vi "Fade Overlay.vi"(11 "Stop Fade":refnum<user-event>) -> ()   [LabVIEW 2020]
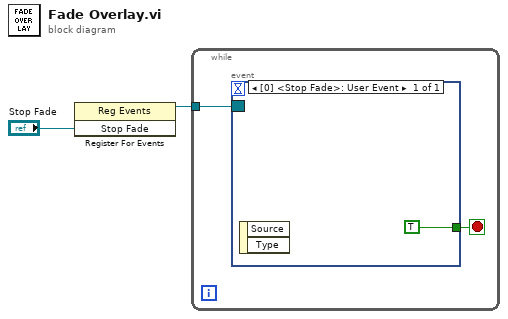
[diagram p0: block diagram]
diagram:
  n1 = register-events("Stop Fade") -> (reference out=w2:refnum<event-registration>)  [unwired: 2 in, 1 out]
  n2 = while {
    tunnel: w2 -> [w4]
    stop <- w3 stop-if-true
    n3 = event shown="[0] <Stop Fade>: User Event" {
      selector: w4 -> [_]
      dyn-events: _ -> [_]
      timeout: _ -> [_]
      tunnel: [TRUE] -> w3
      event User Event {
        n4 = event-data() -> ()  [unwired: 1 in, 2 out]
      }
    }
  }
